vi "sandbox.vi"() -> ()   [LabVIEW 2019, in "ConfigJSON.lvclass"]
uses:
  ConfigJSON.lvclass
  ConfigJSON.lvclass/ConfigJSON.ctl
  c5c0a7b0-2ba1-4883-a31a-00965e90ceef.vi
  <vilib>/Utility/error.llb/Clear Errors.vi
panel:
  out "data":T1
  out "Created":bool
  out "error out":errorcluster
  in  "Config Dir":path
  in  "Cluster":T1 {"Cluster"."Slide" scale=0.0..10.0}
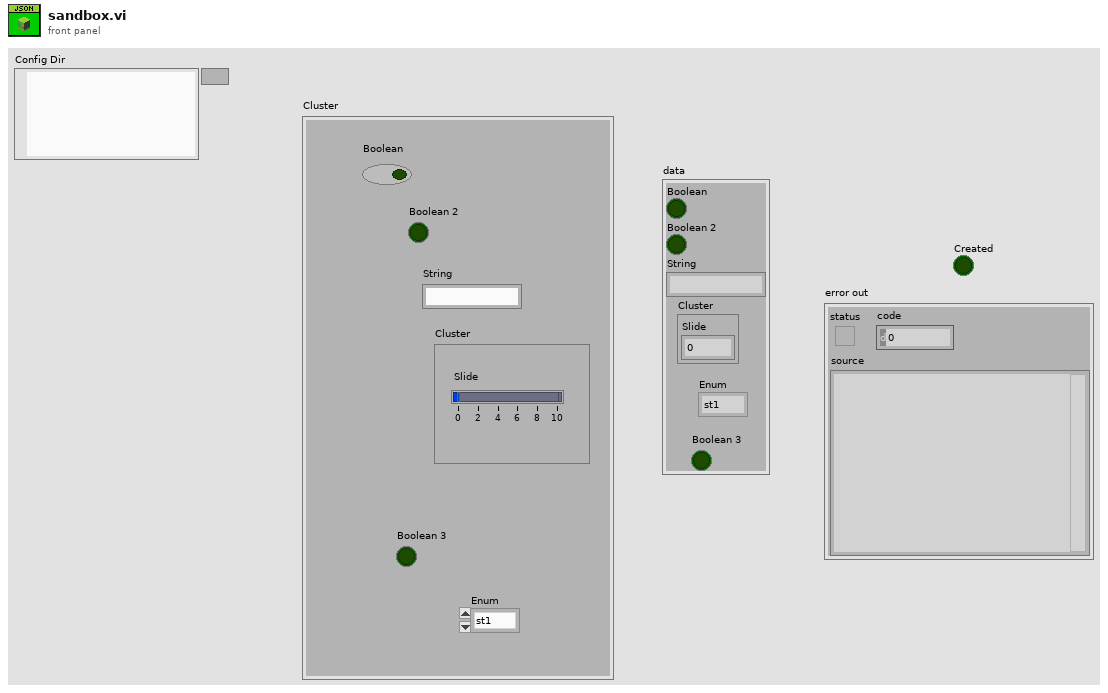
[diagram p1: front panel]
types:
  T1 = cluster{"Boolean":bool, "Boolean 2":bool, "String":string, "Cluster":cluster{"Slide":dbl}, "Boolean 3":bool, "Enum":enum16{"st1", "st2"}}
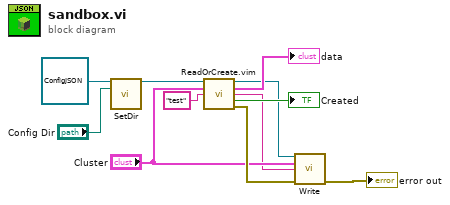
[diagram p0: block diagram]
diagram:
  n1 = call "SetDir.vi"("reference in"=refnum<class "ConfigJSON.lvclass"> refnum ("ConfigJSON"), "Config Dir"="Config Dir") -> ("JSON"=w11:refnum<class "ConfigJSON.lvclass">)  [unwired: 13 in]
  n2 = call "ReadOrCreate.vim"("reference in"=w11, "Type and Defaults"="Cluster", "Name"="test") -> ("reference out"=w5:refnum<class "ConfigJSON.lvclass">, "Data"=→"data":T1, "Name dub"=w2:string, "Created"=→"Created":bool, "error out"=w7:errorcluster)  [unwired: 8 in]
  n3 = call-dynamic "Write.vi"("reference in"=w5, "Data"="Cluster", "Name"=w2, "error in (no error)"=w7) -> ("error out"=→"error out":errorcluster)  [unwired: 8 in, 3 out]
